vi "CH VC simplifiseret v2.vi"() -> ()   [LabVIEW 2022 SP3]
uses:
  <vilib>/vision/driver/NI_Vision_Acquisition_Software.lvlib
  <vilib>/userdefined/High Color/IMAQdx.ctl
panel:
  out "Number of objects":i32
  out "Insect-data-array":dbl[][](array[numeric])
  in  "?":T1(tab)
  in  "Training image on/off":bool
  out "Image from camera/traning image":T2(plugin-control)
  out "Image from vision assistant":T2(plugin-control)
  in  "?":T3(tab)
  out "Objects after sorting":string[][](array[string])
  out "Obejcts after smallest removed":string[][](array[string])
  out "Objects after out of range removed":string[][](array[string])
  out "Initial number of insects":i32
  out "Length of largest insect from\nlatest computer vision picture":dbl
  out "Number of insects after smallest specified removed":i32
  out "Number of insects after out of range removed":i32
  out "Loop number":i32
  out "Errosion number":i32
  out "Match Score (Color Matching 1)":i32[](array[numeric])
  out "Black image error":bool
  in  "Stop program":bool
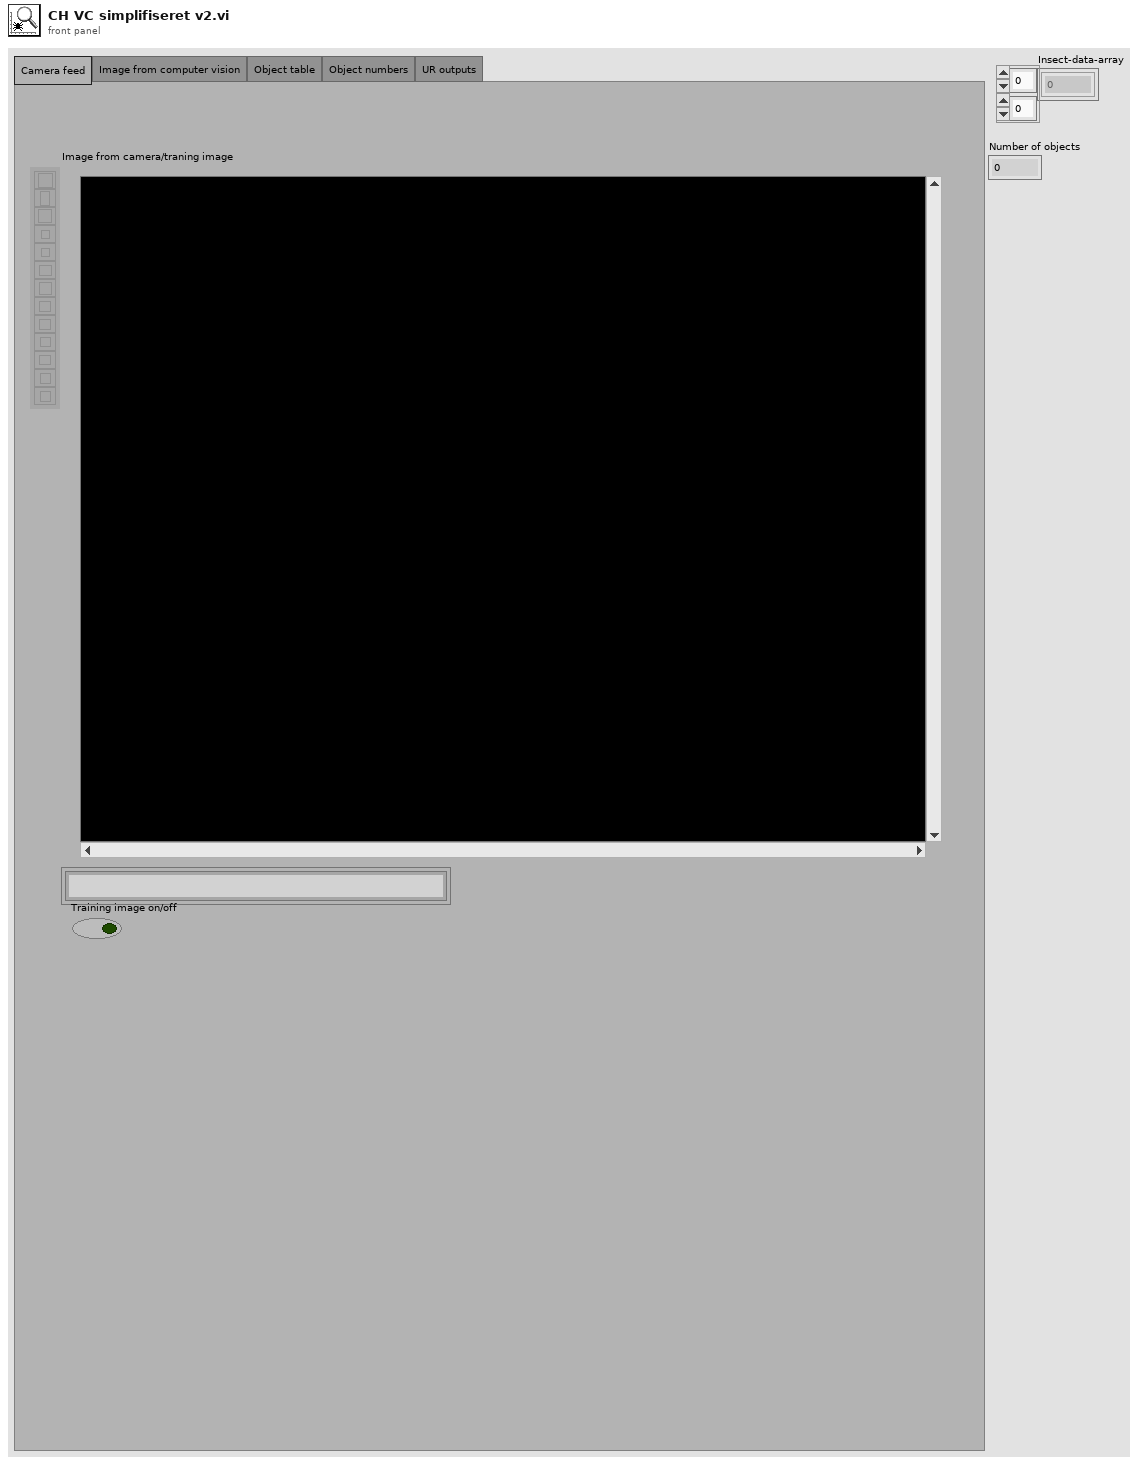
[diagram p1: front panel]
types:
  T1 = enum32{"Camera feed", "Image from computer vision", "Object table", "Object numbers", "UR outputs"}
  T2 = typedef "IMAQ Image.ctl" = refnum<image>
  T3 = enum32{"Objects after sorting", "Objects after smallest removed", "Objects after out of range removed"}
  T4 = typedef "Image Type" = u32
  T5 = typedef "IMAQdx.ctl" = refnum<k21>
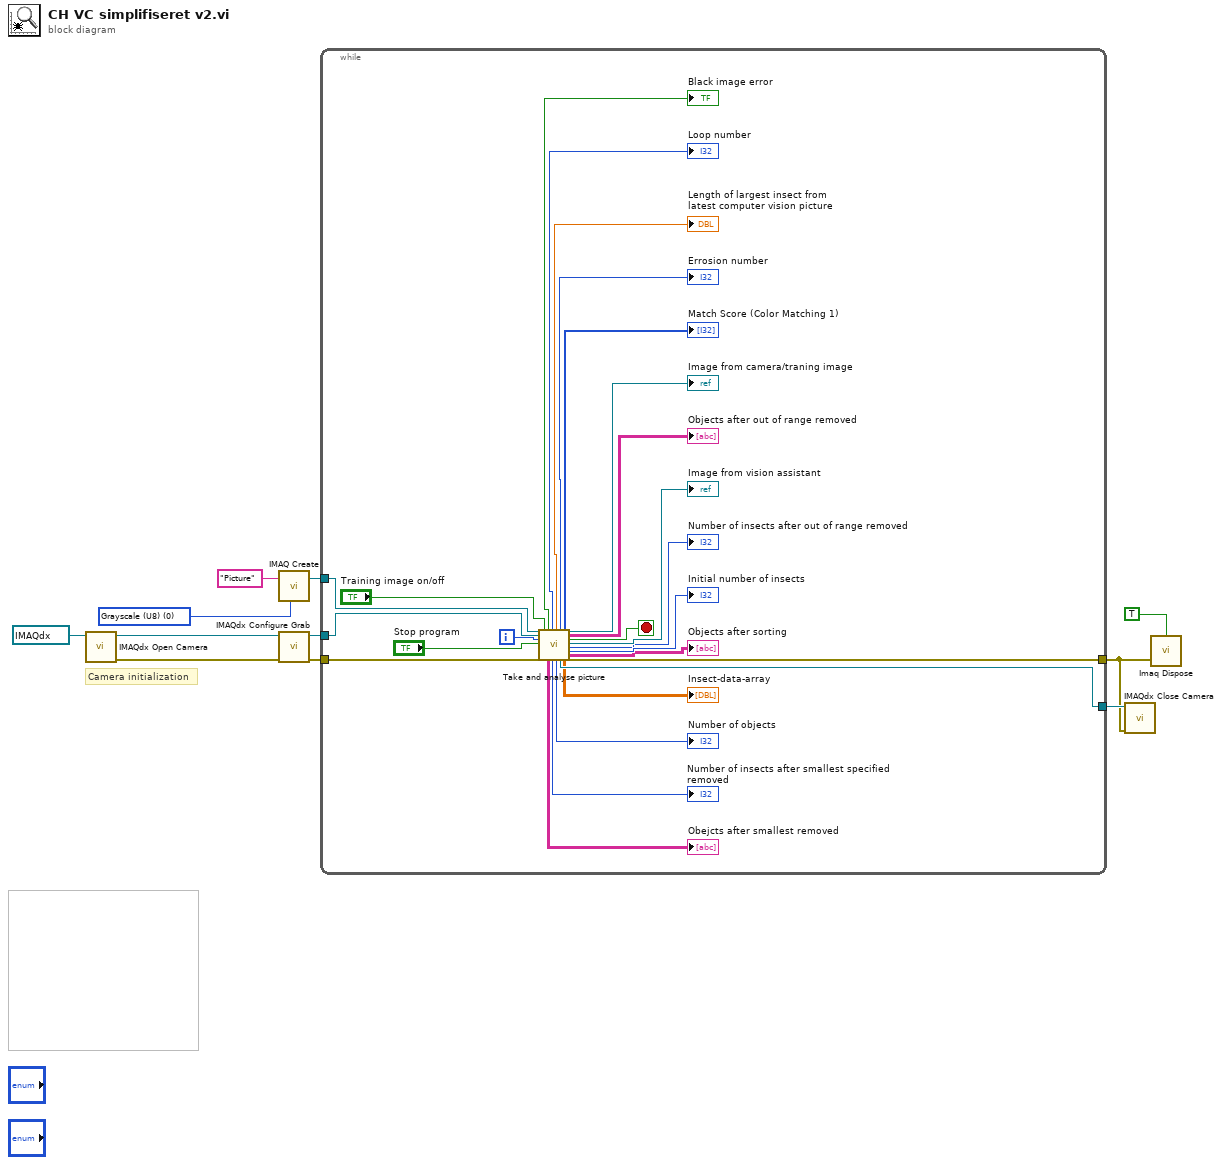
[diagram p0: block diagram]
diagram:
  w3 = T4 0 items=["Grayscale (U8)", "Grayscale (I16)", "Grayscale (SGL)", "Complex (CSG)", "RGB (U32)", "HSL (U32)", "RGB (U64)", "Grayscale (U16)"] ("Image Type")
  # "Camera initialization"
  n1 = call <vilib>:"IMAQdx Open Camera.vi"("Session In"=T5 "cam2") -> ("error out"=w4:errorcluster, "Session Out"=w8:T5)  [unwired: 9 in]
  n2 = call "IMAQ Create"("Image Name"="Picture", "Image Type"=w3) -> ("New Image"=w10:T2)  [unwired: 3 in, 1 out]
  n3 = call <vilib>:"IMAQdx Configure Grab.vi"("error in"=w4, "Session In"=w8) -> ("error out"=w5:errorcluster, "Session Out"=w7:T5)  [unwired: 8 in]
  n4 = while {
    tunnel: w10 -> [w33]
    tunnel: w7 -> [w35]
    tunnel: [w32] -> w6
    tunnel: [w26] -> w2
    tunnel: w5 -> [w34]
    i -> [w31]
    stop <- w28 stop-if-true
    n5 = call "Take and analyse picture.vi"("Refnum in"=w33, "Session Out in"=w35, "Numeric"=w31, "Stop program"="Stop program", "error in (no error)"=w34, "Training image on/off"="Training image on/off") -> ("Black image error"=→"Black image error":bool, "Obejcts after smallest removed"=→"Obejcts after smallest removed":string[][], "Loop number"=→"Loop number":i32, "Number of insects after smallest specified removed"=→"Number of insects after smallest specified removed":i32, "Length of largest insect from\nlatest computer vision picture"=→"Length of largest insect from\nlatest computer vision picture":dbl, "Number of objects"=→"Number of objects":i32, "Errosion number"=→"Errosion number":i32, "Session Out out"=w32:T5, "Match Score (Color Matching 1)"=→"Match Score (Color Matching 1)":i32[], "Insect-data-array (out of range removed)"=→"Insect-data-array":dbl[][], "Refnum out"=→"Image from camera/traning image":T2, "Objects after out of range removed"=→"Objects after out of range removed":string[][], "Boolean"=w28:bool, "Image from vision assistant"=→"Image from vision assistant":T2, "Number of insects after out of range removed"=→"Number of insects after out of range removed":i32, "Initial number of insects"=→"Initial number of insects":i32, "Objects after sorting"=→"Objects after sorting":string[][], "error out"=w26:errorcluster)  [unwired: 4 in]
  }
  n6 = call <vilib>:"IMAQdx Close Camera.vi"("error in"=w2, "Session In"=w6) -> ()  [unwired: 9 in, 1 out]
  n7 = call "Imaq Dispose"("All Images? (No)"=TRUE, "error in (no error)"=w2) -> ()  [unwired: 4 in, 1 out]
